vi "Register Indicator.vi"(8 "error in (no error)":errorcluster, 10 "GUI Element":refnum<class "GUI Element.lvclass">, 11 "PluginGUI in":refnum<class "PluginGUI.lvclass">) -> (0 "error out":errorcluster, 3 "PluginGUI out":refnum<class "PluginGUI.lvclass">)   [LabVIEW 2020, in "VolatusGUI.lvlib" / "PluginGUI.lvclass"]
uses:
  PluginGUI.lvclass
  GUI Element/GUI Element.lvclass
  Indicator/Indicator.lvclass
  C:/dev/lv20CE/relink/lv-volatus/VolatusGUI/GUI Element/GUI Element.lvclass
  PluginGUI.lvclass/PluginGUI.ctl
  GUI Element/GUI Element.lvclass/GUI Element.ctl
  C:/dev/lv20CE/relink/lv-volatus/VolatusGUI/Indicator/Indicator.lvclass
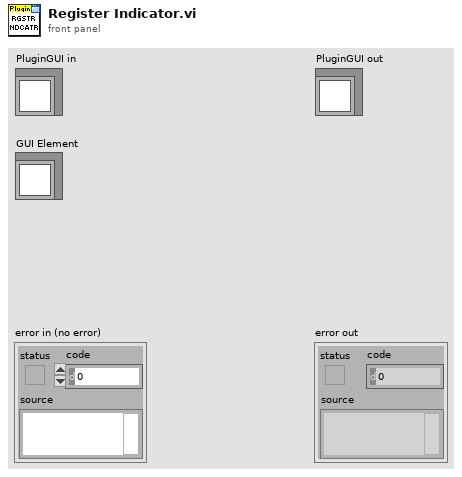
[diagram p1: front panel]
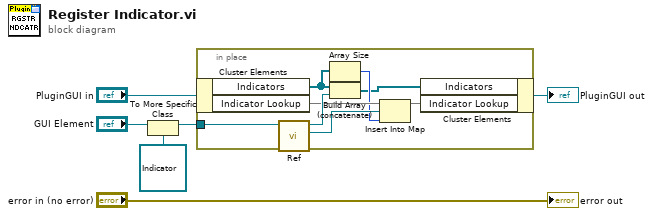
[diagram p0: block diagram]
diagram:
  n1 = To More Specific Class(target class=refnum<class "Indicator.lvclass"> refnum ("VolatusGUI:Indicator"), reference="GUI Element") -> (specific class reference=w2:refnum<class "Indicator.lvclass">)  [unwired: 1 in, 1 out]
  n2 = in-place {
    in-place-border: w2 -> [w14]
    n3 = in-place-cluster #1("PluginGUI in") -> ("Indicators"=w13:refnum<class "Indicator.lvclass">[], "Indicator Lookup"=w11:map{refnum<vi>, i32})
    n4 = call "Ref.vi"("GUI Element in"=w14) -> ("Ref"=w10:refnum<vi>, "GUI Element out"=w12:refnum<class "Indicator.lvclass">)  [unwired: 9 in]
    n5 = Array Size(array=w13) -> (size(s)=w9:i32)
    n6 = Build Array (concatenate)(w13, w12) -> (w7:refnum<class "Indicator.lvclass">[])
    n7 = Insert Into Map(map in=w11, key=w10, value=w9) -> (map out=w8:map{refnum<vi>, i32})  [unwired: 2 out]
    n8 = in-place-cluster #1("Indicators"=w7, "Indicator Lookup"=w8) -> (→"PluginGUI out":refnum<class "PluginGUI.lvclass">)
  }
  "error out" <- "error in (no error)"
